vi "AD7609_SampleDual.vi"() -> (0 "OK":bool, 1 "FRSTDATA 2":bool[](array[boolean]), 2 "FRSTDATA":bool[](array[boolean]), 3 "DATA":i16[](array[numeric])=[9827, -1, 0, -1, -1, 1, 3, 13138, 0, 0, 0, 0, 0, 0, 0, 0])   [LabVIEW 2012]
uses:
  glADC.vi
  <vilib>/rvi/eio/common/nirviEmuTemplateMethod_errors.vi
  <vilib>/eio/EIONode/EIONode.xnode
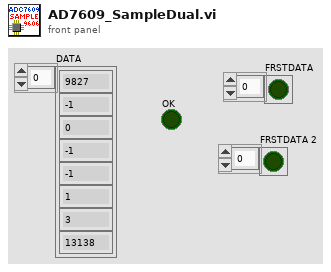
[diagram p1: front panel]
types:
  T1 = cluster{"OS":u8, "Range":u8, "T_hi":u8, "D_low":u8}
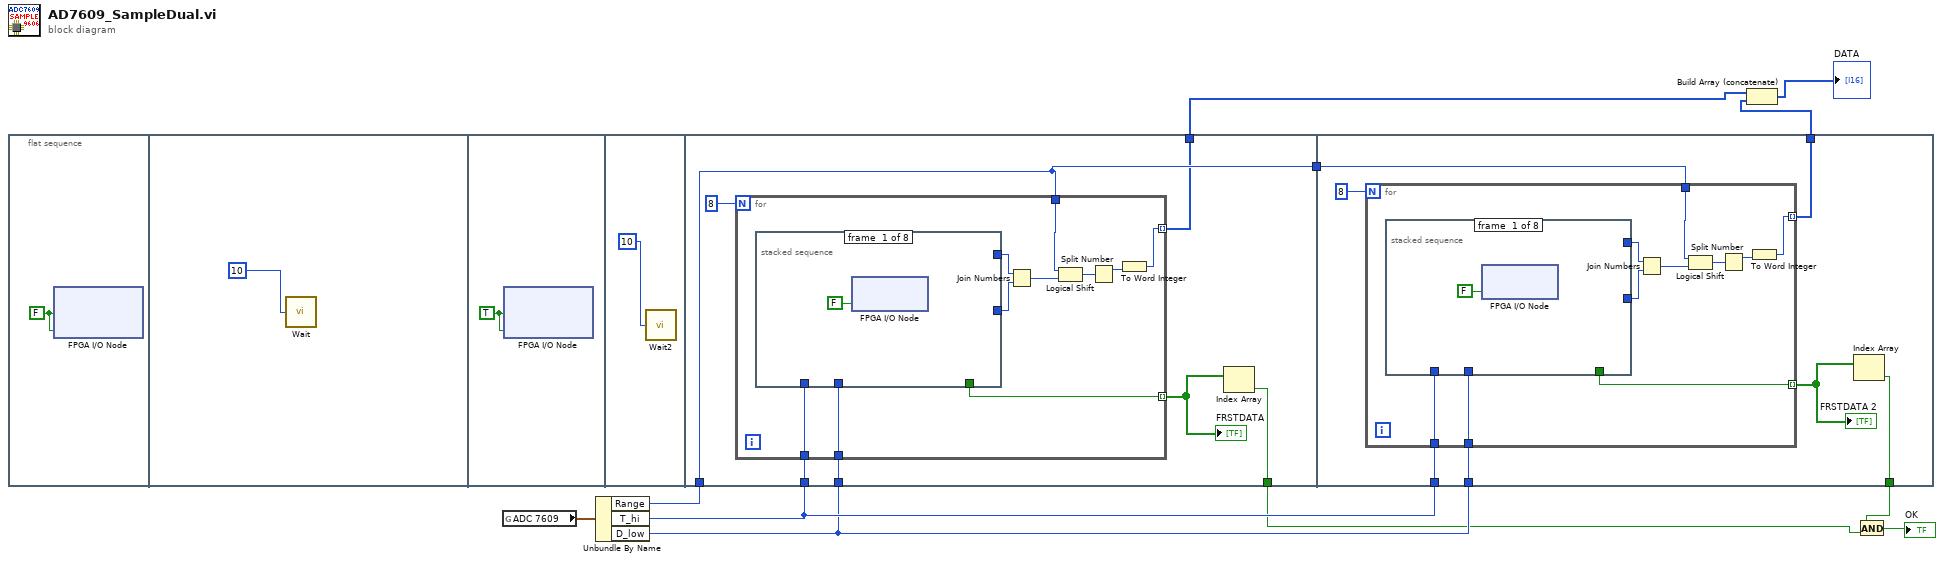
[diagram p0: block diagram]
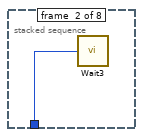
[diagram p2: hidden frame]
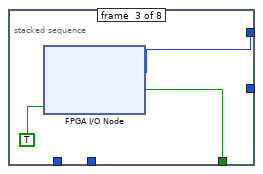
[diagram p3: hidden frame]
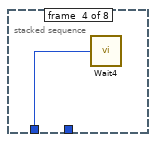
[diagram p4: hidden frame]
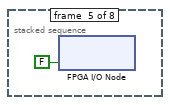
[diagram p5: hidden frame]
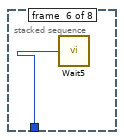
[diagram p6: hidden frame]
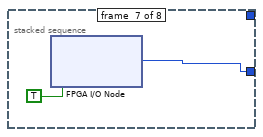
[diagram p7: hidden frame]
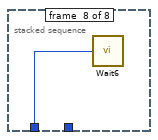
[diagram p8: hidden frame]
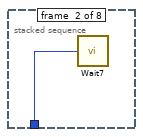
[diagram p9: hidden frame]
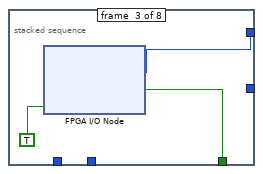
[diagram p10: hidden frame]
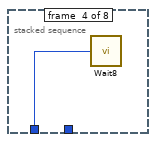
[diagram p11: hidden frame]
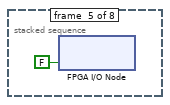
[diagram p12: hidden frame]
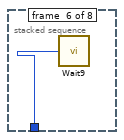
[diagram p13: hidden frame]
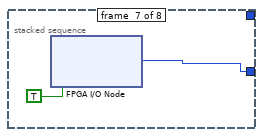
[diagram p14: hidden frame]
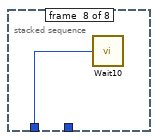
[diagram p15: hidden frame]
diagram:
  n1 = flat-sequence {
    tunnel: w7 -> [w21]
    tunnel: w8 -> [w20]
    tunnel: w10 -> [w18]
    tunnel: [w18] -> w9
    tunnel: [w17] -> w5
    tunnel: [w16] -> w1
    tunnel: w9 -> [w48]
    tunnel: w8 -> [w47]
    tunnel: w7 -> [w46]
    tunnel: [w45] -> w4
    tunnel: [w44] -> w2
    frame #0 {
      w12 = FALSE ("RESET")
      n2 = xnode "FPGA I/O Node"("CONVST1"=w12, "CONVST2"=w12) -> ()  [unwired: 2 in, 2 out]
    }
    frame #1 {
      n3 = call "Wait"("Count(Ticks)"=u8 10 ("T_convst")) -> ()  [unwired: 1 out]
    }
    frame #2 {
      w14 = TRUE ("RESET")
      n4 = xnode "FPGA I/O Node"("CONVST1"=w14, "CONVST2"=w14) -> ()  [unwired: 2 in, 2 out]
    }
    frame #3 {
      n5 = call "Wait2"("Count(Ticks)"=u8 10 ("D_convst")) -> ()  [unwired: 1 out]
    }
    frame #4 {
      n6 = for {
        N: 8 -> [_]
        tunnel: [w24] -> w17 mode=indexing
        tunnel: [w32] -> w19 mode=indexing
        tunnel: w21 -> [w31]
        tunnel: w20 -> [w30]
        tunnel: w18 -> [w23]
        n7 = stacked-sequence {
          tunnel: [_ _ w35 _ _ _ _ _] -> w29
          tunnel: [_ _ w37 _ _ _ _ _] -> w32
          tunnel: [_ _ _ _ _ _ w41 _] -> w28
          tunnel: w31 -> [_ w34 _ _ _ w40 _ _]
          tunnel: w30 -> [_ _ _ w38 _ _ _ w43]
          frame #0 {
            n8 = xnode "FPGA I/O Node"("RD1"=FALSE ("RD")) -> ()  [unwired: 1 in, 1 out]
          }
          frame #1 {
            n9 = call "Wait3"("Count(Ticks)"=w34) -> ()  [unwired: 1 out]
          }
          frame #2 {
            n10 = xnode "FPGA I/O Node"("RD1"=TRUE ("RD")) -> ("DB0-DB15"=w35:u16, "FRSTDATA1"=w37:bool)  [unwired: 3 in, 3 out]
          }
          frame #3 {
            n11 = call "Wait4"("Count(Ticks)"=w38) -> ()  [unwired: 1 out]
          }
          frame #4 {
            n12 = xnode "FPGA I/O Node"("RD1"=FALSE ("RESET")) -> ()  [unwired: 1 in, 1 out]
          }
          frame #5 {
            n13 = call "Wait5"("Count(Ticks)"=w40) -> ()  [unwired: 1 out]
          }
          frame #6 {
            n14 = xnode "FPGA I/O Node"("RD1"=TRUE ("RD")) -> ("DB0-DB15"=w41:u16)  [unwired: 2 in, 2 out]
          }
          frame #7 {
            n15 = call "Wait6"("Count(Ticks)"=w43) -> ()  [unwired: 1 out]
          }
        }
        n16 = Join Numbers(hi=w29, lo=w28) -> ((hi.lo)=w27:u32)
        n17 = Logical Shift(y=w23, x=w27) -> (x << y=w26:u32)
        n18 = Split Number(x=w26) -> (hi(x)=w25:u16)  [unwired: 1 out]
        n19 = To Word Integer(number=w25) -> (16bit integer=w24:i16)
      }
      "FRSTDATA" <- w19
      n20 = Index Array(array=w19) -> (element=w16:bool)  [unwired: 1 in]
    }
    frame #5 {
      n21 = for {
        N: 8 -> [_]
        tunnel: [w52] -> w45 mode=indexing
        tunnel: [w60] -> w50 mode=indexing
        tunnel: w46 -> [w59]
        tunnel: w47 -> [w58]
        tunnel: w48 -> [w51]
        n22 = stacked-sequence {
          tunnel: [_ _ w63 _ _ _ _ _] -> w57
          tunnel: [_ _ w65 _ _ _ _ _] -> w60
          tunnel: [_ _ _ _ _ _ w69 _] -> w56
          tunnel: w59 -> [_ w62 _ _ _ w68 _ _]
          tunnel: w58 -> [_ _ _ w66 _ _ _ w71]
          frame #0 {
            n23 = xnode "FPGA I/O Node"("RD2"=FALSE ("RD")) -> ()  [unwired: 1 in, 1 out]
          }
          frame #1 {
            n24 = call "Wait7"("Count(Ticks)"=w62) -> ()  [unwired: 1 out]
          }
          frame #2 {
            n25 = xnode "FPGA I/O Node"("RD2"=TRUE ("RD")) -> ("DB0-DB15"=w63:u16, "FRSTDATA2"=w65:bool)  [unwired: 3 in, 3 out]
          }
          frame #3 {
            n26 = call "Wait8"("Count(Ticks)"=w66) -> ()  [unwired: 1 out]
          }
          frame #4 {
            n27 = xnode "FPGA I/O Node"("RD2"=FALSE ("RESET")) -> ()  [unwired: 1 in, 1 out]
          }
          frame #5 {
            n28 = call "Wait9"("Count(Ticks)"=w68) -> ()  [unwired: 1 out]
          }
          frame #6 {
            n29 = xnode "FPGA I/O Node"("RD2"=TRUE ("RD")) -> ("DB0-DB15"=w69:u16)  [unwired: 2 in, 2 out]
          }
          frame #7 {
            n30 = call "Wait10"("Count(Ticks)"=w71) -> ()  [unwired: 1 out]
          }
        }
        n31 = Join Numbers(hi=w57, lo=w56) -> ((hi.lo)=w55:u32)
        n32 = Logical Shift(y=w51, x=w55) -> (x << y=w54:u32)
        n33 = Split Number(x=w54) -> (hi(x)=w53:u16)  [unwired: 1 out]
        n34 = To Word Integer(number=w53) -> (16bit integer=w52:i16)
      }
      "FRSTDATA 2" <- w50
      n35 = Index Array(array=w50) -> (element=w44:bool)  [unwired: 1 in]
    }
  }
  n36 = global read "glADC.vi" "ADC 7609"() -> (w11:T1)
  n37 = Unbundle By Name(w11) -> ("Range"=w10:u8, "T_hi"=w8:u8, "D_low"=w7:u8)
  n38 = Build Array (concatenate)(w5, w4) -> (→"DATA":i16[])
  n39 = And(x=w2, y=w1) -> (x .and. y?=→"OK":bool)
